vi "Varian Max Field.vi"() -> ()   [LabVIEW 2009, in "Varian Magnet.lvclass"]
uses:
  Varian Magnet.lvclass
panel:
  in  "Varian Max Field":dbl[unit]=0.8
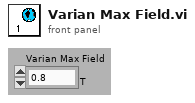
[diagram p1: front panel]
diagram:
